vi "PackASCIIString.vi"(8 "Error In":errorcluster, 11 "string":string="MFC-1234") -> (0 "Error Out":errorcluster, 3 "Packed Byte Array":u8[](array[numeric])=[52, 96, 237, 199, 44, 244] format="%x")   [LabVIEW 2016, in "Brooks MFC.lvclass"]
doc: "Reconstruction of ASCII characters from Packed (6bist ASCII) data format"
uses:
  Brooks MFC.lvclass
panel:
  out "Array":bool[][](array[boolean])
  # "Example: \n(Hex) 34 60 ED   C7 2C F4\ntransforms to \"MFC-1234\""
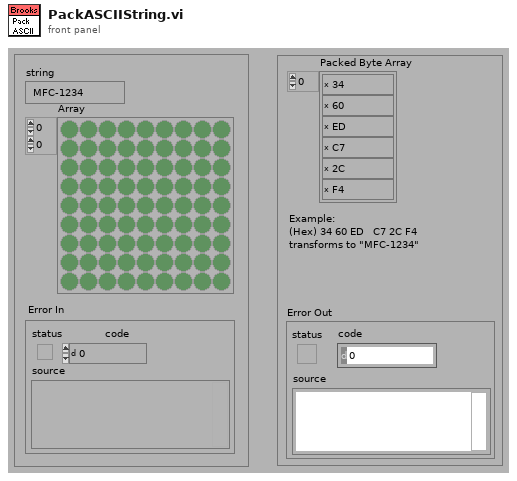
[diagram p1: front panel]
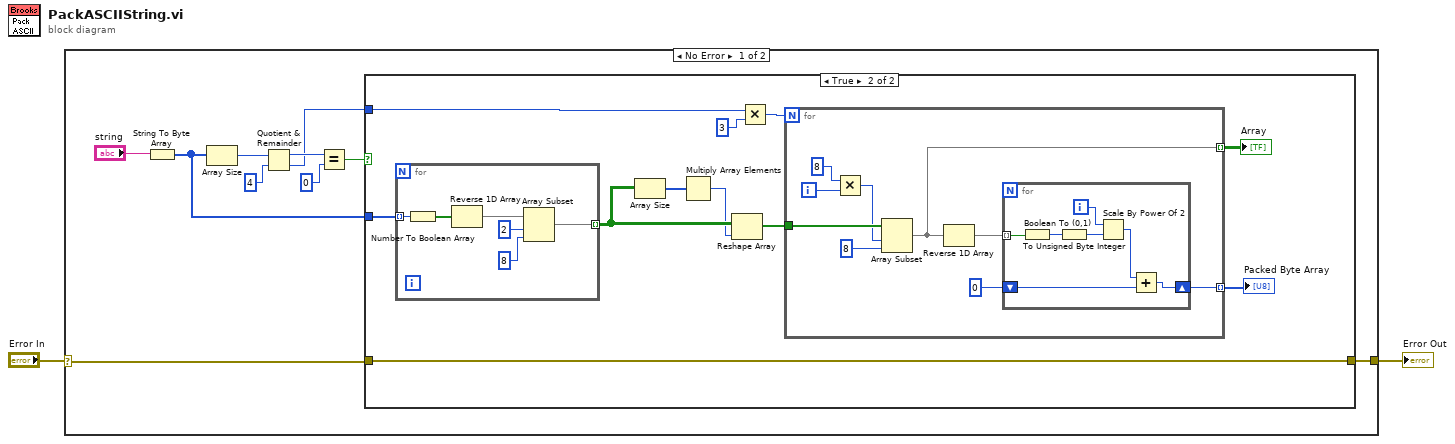
[diagram p0: block diagram]
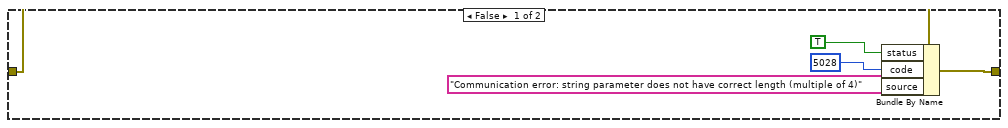
[diagram p2: hidden frame]
diagram:
  n1 = case shown="No Error" "Error In" {
    selector: "Error In" -> [w3 w51]
    tunnel: [w4 w51] -> w2
    frame No Error {
      n2 = String To Byte Array(string="string") -> (unsigned byte array=w5:u8[])
      n3 = Array Size(array=w5) -> (size(s)=w12:i32)
      n4 = Quotient & Remainder(x=w12, y=4) -> (x-y*floor(x/y)=w10:i32, floor(x/y)=w7:i32)
      n5 = Equal?(x=w10, y=0) -> (x = y?=w8:bool)
      n6 = case shown="True" w8 {
        tunnel: w7 -> [_ w27]
        tunnel: w5 -> [_ w26]
        tunnel: w3 -> [w17 w18]
        tunnel: [w16 w18] -> w4
        frame False {
          n7 = Bundle By Name(cluster=w17, "status"=TRUE, "code"=5028, "source"="Communication error: string parameter does not have correct length (multiple of 4)") -> (w16:errorcluster)
        }
        frame True {
          n8 = for {
            tunnel: w26 -> [w49] mode=indexing
            tunnel: [w45] -> w25 mode=indexing
            n9 = Number To Boolean Array(number=w49) -> (Boolean array=w50:bool[])
            n10 = Reverse 1D Array(array=w50) -> (reversed array=w48:bool[])
            n11 = Array Subset(array=w48, index=2, length=8) -> (w45:bool[])
          }
          n12 = Array Size(array=w25) -> (size(s)=w24:i32[])
          n13 = Multiply Array Elements(1:w24) -> (0:w23:i32)
          n14 = Reshape Array(w25, w23) -> (w22:bool[])
          n15 = Multiply(x=w27, y=i16 3) -> (x*y=w21:i32)
          n16 = for {
            N: w21 -> [_]
            tunnel: w22 -> [w37]
            tunnel: [w31] -> w20 mode=indexing
            tunnel: [w30] -> w19 mode=indexing
            i -> [w34]
            n17 = Multiply(x=8, y=w34) -> (x*y=w35:i32)
            n18 = Array Subset(array=w37, index=w35, length=8) -> (w30:bool[])
            n19 = Reverse 1D Array(array=w30) -> (reversed array=w29:bool[])
            n20 = for {
              shift-right: [w41] -> w31
              shift-left: u8 0 -> [w42]
              tunnel: w29 -> [w38] mode=indexing
              i -> [w39]
              n21 = Boolean To (0,1)(Boolean=w38) -> (0, 1=w44:i16)
              n22 = To Unsigned Byte Integer(number=w44) -> (unsigned 8bit integer=w40:u8)
              n23 = Scale By Power Of 2(n=w39, x=w40) -> (x*2^n=w43:u8)
              n24 = Add(x=w43, y=w42) -> (x+y=w41:u8)
            }
          }
          "Packed Byte Array" <- w20
          "Array" <- w19
        }
      }
    }
    frame Error {
    }
  }
  "Error Out" <- w2
